vi "PWA_Setup_Panel.vi"(0 "Show Panel?":bool, 1 "Check Calib file?":bool, 2 "OK":T1, 3 "Incoming Setup String":string) -> (7 "Outgoing Setup String":string)   [LabVIEW 2017]
uses:
  Controls/ok_button.ctl
  File/Setup_Filetype.ctl
  Controls/Post_Process.ctl
  Controls/App_Global.ctl
  Controls/Inst_type.ctl
  Globals/Meas_global.vi
  PWAtasksGLOBAL.vi
panel:
  in  "Probe Rotated Thro' 180":bool
  in  "Software + buffering delay per pulse (s)":dbl=9.7e-06
  in  "Symbol":string
  in  "Pulse length \nx2 micro sec":i16=1 min=1 max=12
  in  "Clock Rate":bool
  in  "Gain":i16=1 min=1 max=12
  in  "Wire Current mA":i16(knob)=1 min=1 max=3 step=1 scale=1.0..3.0
  in  "Trigger -ve":dbl(knob)=1.0 min=0.0 max=5.0 scale=0.0..5.0 scale format="%#.2f"
  in  "Trigger +ve":dbl(knob)=1.0 min=0.0 max=5.0 scale=0.0..5.0 scale format="%#.2f"
  out "Calib Path from file":path
  in  "Use Latest":bool=TRUE
  in  "PWA Calib. File Path":path=path "/G5_1_HD/Users/paulhayden/Desktop/Labview test/PWA_Calib.xls"
  in  "Minimum TOF (mu.s)":i16=225
  in  "PWA Freq. (Hz)":dbl=30.0 min=0.0 max=50.0
  # "PELA Flow Instruments Ltd."
  # "TRIGGER LEVELS\n(volts)"
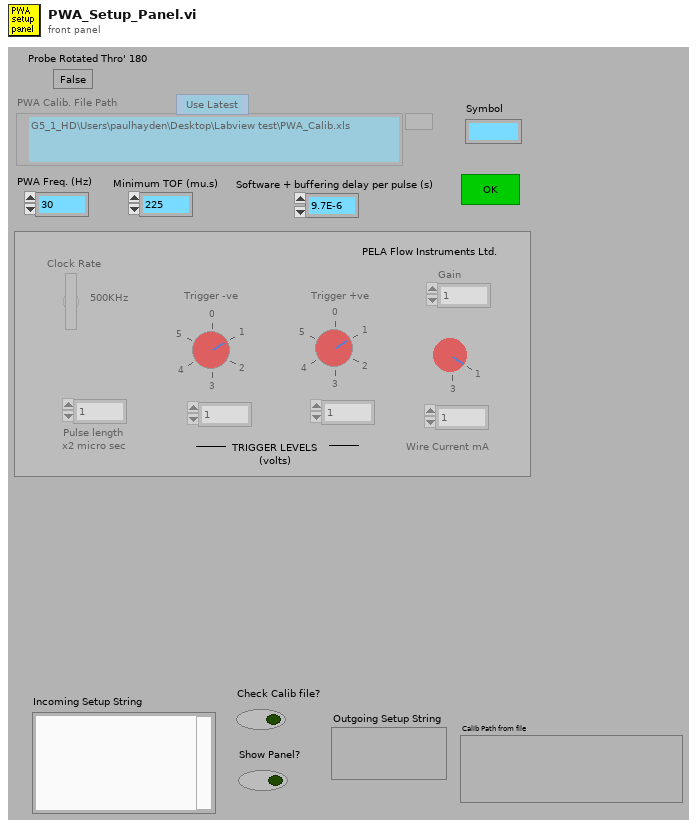
[diagram p1: front panel]
types:
  T1 = typedef "ok_button.ctl" = bool
  T2 = typedef "Setup_Filetype.ctl" = enum16{"Measurement Setups", "Calibration Setups", "General", "Results File Plotter Setups", "Speed Calib Tweaks"}
  T3 = typedef "Post_Process.ctl" = enum16{"Take New Data", "Post Process Raw Data File"}
  T4 = typedef "App_Global.ctl" = enum16{"Read Global", "Write to Global", "Initialise Array"}
  T5 = typedef "Inst_type.ctl" = enum16{"Propeller anemometer", "Raw voltage", "Pressure Transducer", "Pitot-static tube", "Preston tube", "Hot wire", "Cross wire 1", "Cross wire 2", "Generic Linear", "Generic Polynomial", "Generic BackPoly", "Fast FID", "Thermocouple", "Cold wire", "Pulsed Wire", "LDA Vel", "LDA Tran time", "LDA Arr time", "Microphone"}
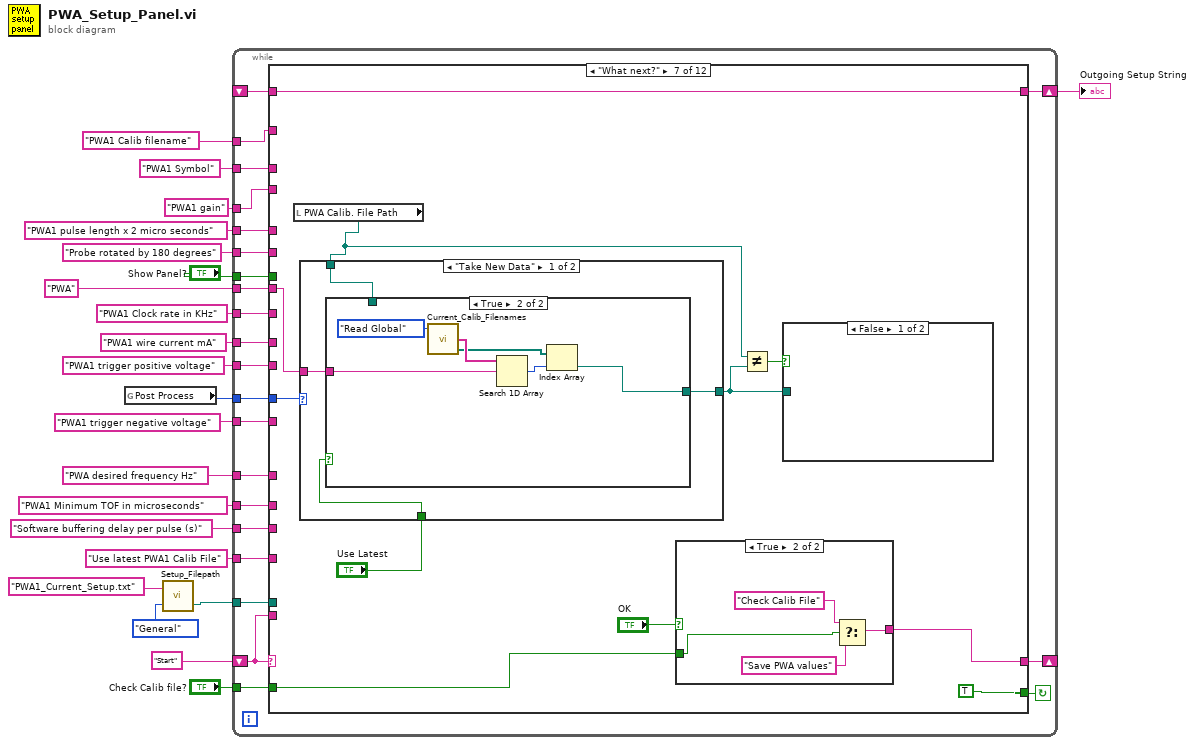
[diagram p0: block diagram]
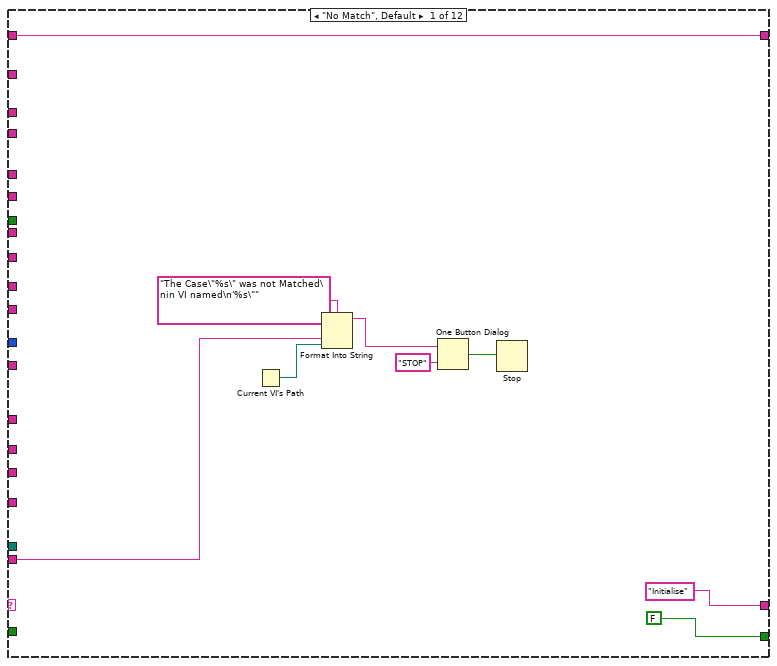
[diagram p2: hidden frame]
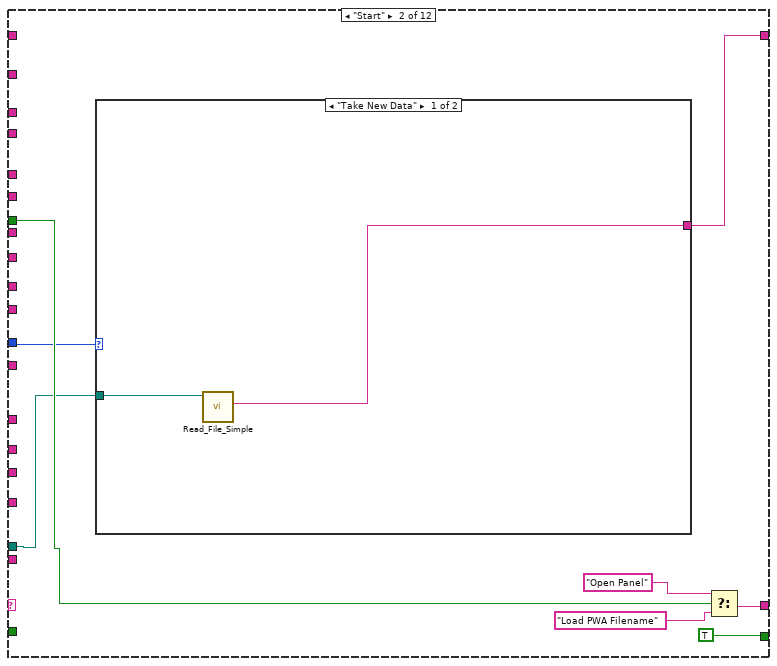
[diagram p3: hidden frame]
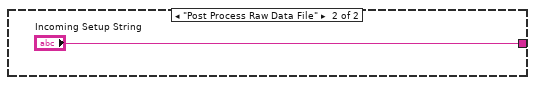
[diagram p4: hidden frame]
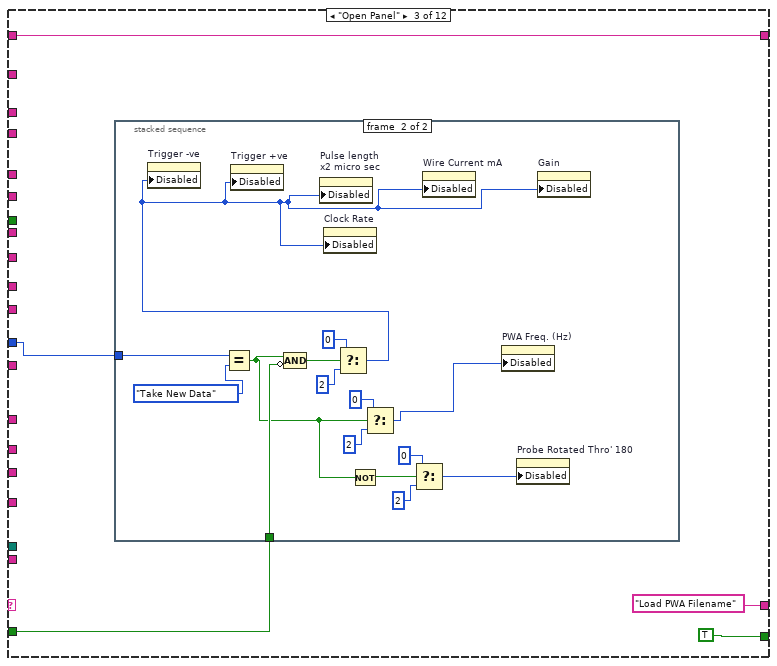
[diagram p5: hidden frame]
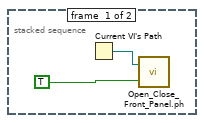
[diagram p6: hidden frame]
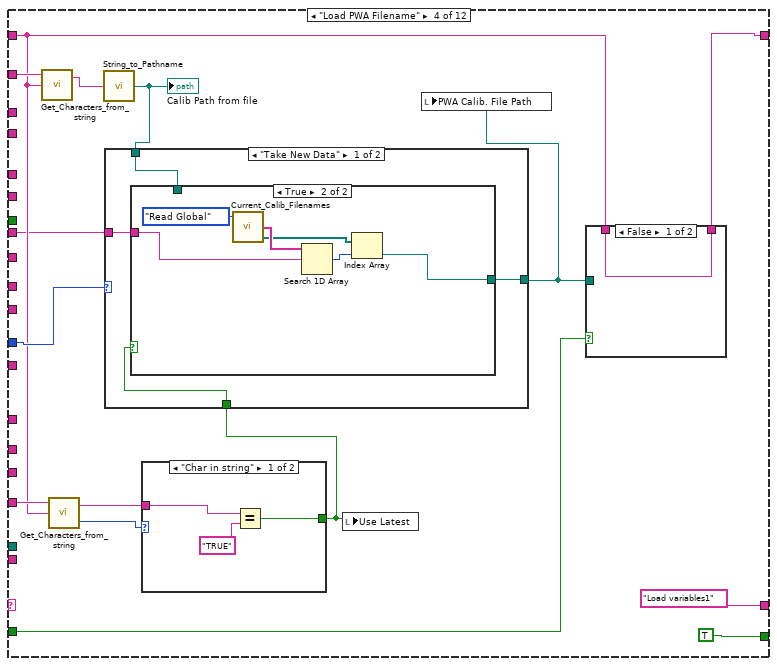
[diagram p7: hidden frame]
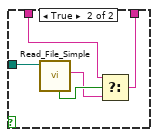
[diagram p8: hidden frame]
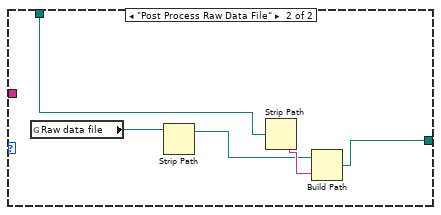
[diagram p10: hidden frame]
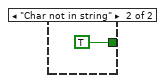
[diagram p11: hidden frame]
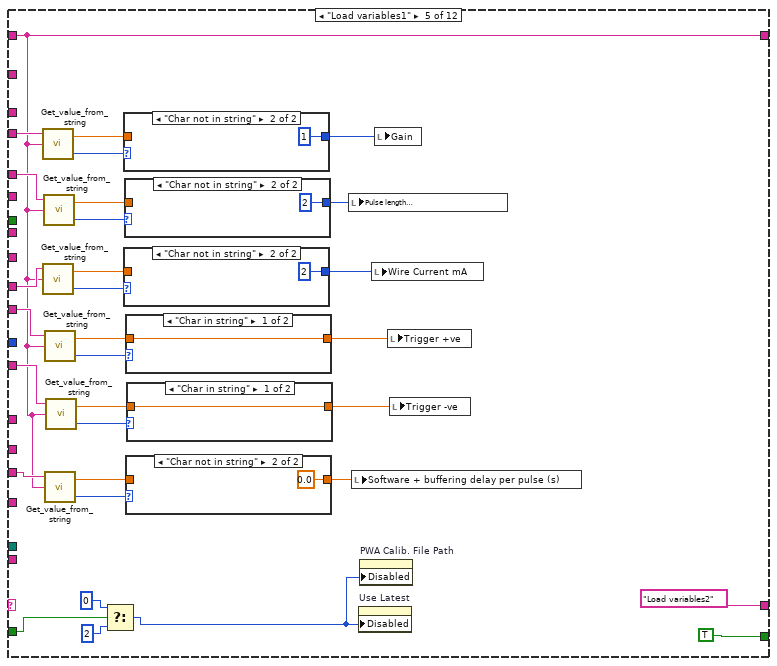
[diagram p12: hidden frame]
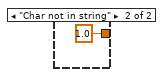
[diagram p14: hidden frame]
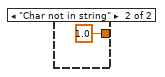
[diagram p15: hidden frame]
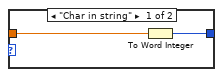
[diagram p16: hidden frame]
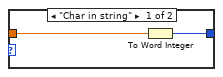
[diagram p17: hidden frame]
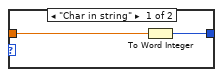
[diagram p18: hidden frame]
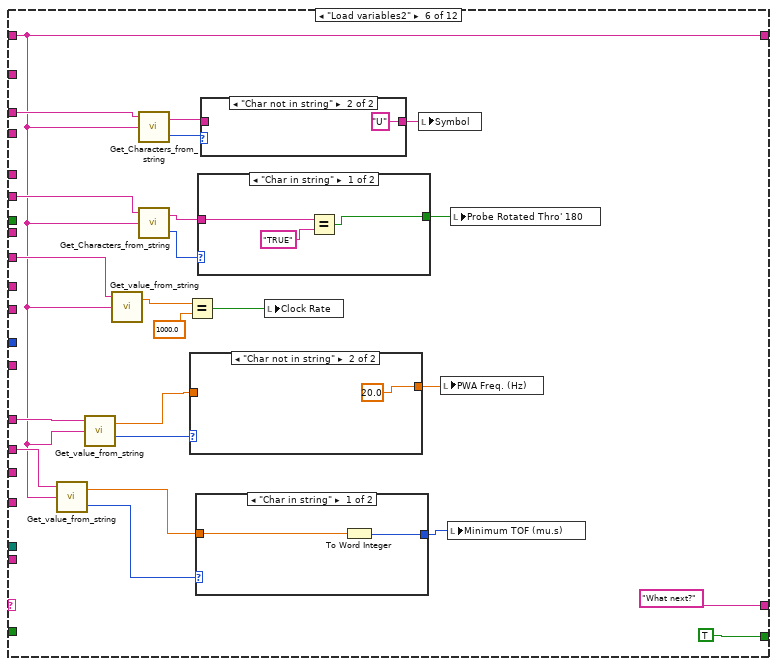
[diagram p19: hidden frame]
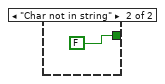
[diagram p20: hidden frame]
diagram:
  n1 = global read "Meas_global.vi" "Post Process"() -> (w20:T3)
  n2 = call "Setup_Filepath.vi"("Setup File Type"=Setup_Filetype."General", "Filename in"="PWA1_Current_Setup.txt" ("name or relative path")) -> ("Filename Out"=w2:path)  [unwired: 1 out]
  n3 = while {
    shift-left: "Start" -> [w43]
    shift-right: [w44] -> _
    tunnel: "Show Panel?" -> [w42]
    tunnel: w20 -> [w41]
    tunnel: "PWA1 Calib filename" -> [w39]
    tunnel: "Use latest PWA1 Calib File" -> [w40]
    tunnel: "PWA1 Minimum TOF in microseconds" -> [w38]
    tunnel: "PWA desired frequency Hz" -> [w37]
    tunnel: "Check Calib file?" -> [w36]
    tunnel: "PWA1 gain" -> [w35]
    tunnel: "PWA1 pulse length x 2 micro seconds" -> [w34]
    tunnel: "PWA1 wire current mA" -> [w33]
    tunnel: "PWA1 trigger positive voltage" -> [w32]
    tunnel: "PWA1 trigger negative voltage" -> [w31]
    tunnel: "PWA1 Clock rate in KHz" -> [w30]
    shift-right: [w29] -> w7
    shift-left: _ -> [w28]
    tunnel: "PWA1 Symbol" -> [w27]
    tunnel: w2 -> [w26]
    tunnel: "Software buffering delay per pulse (s)" -> [w25]
    tunnel: "Probe rotated by 180 degrees" -> [w24]
    tunnel: "PWA" ("element") -> [w23]
    stop <- w45 continue-if-true
    n4 = case shown="\"What next?\"" w43 {
      tunnel: [FALSE TRUE TRUE TRUE TRUE TRUE TRUE TRUE ("Show Panel?") TRUE ("Show Panel?") TRUE ("Show Panel?") w338 FALSE ("Show Panel?")] -> w45
      tunnel: ["Initialise" w55 "Load PWA Filename" "Load variables1" "Load variables2" "What next?" w216 "Save PWA values" "2nd Save PWA values" "PWA Setup Summary" "Close Panel" "End"] -> w44
      tunnel: w43 -> [w49 _ _ _ _ _ _ _ _ _ _ _]
      tunnel: w42 -> [_ w61 _ _ _ _ _ _ _ _ w338 _]
      tunnel: w41 -> [_ w58 w68 w94 _ _ w218 _ _ _ _ w340]
      tunnel: w40 -> [_ _ _ w96 _ _ _ _ w276 _ _ _]
      tunnel: w39 -> [_ _ _ w99 _ _ _ _ w286 _ _ _]
      tunnel: w38 -> [_ _ _ _ _ w195 _ _ w284 _ _ _]
      tunnel: w37 -> [_ _ _ _ _ w194 _ _ w285 _ _ _]
      tunnel: w36 -> [_ _ w66 w91 w157 _ w214 _ _ _ _ _]
      tunnel: w35 -> [_ _ _ _ w150 _ _ _ _ w323 _ _]
      tunnel: w34 -> [_ _ _ _ w146 _ _ _ _ w307 _ _]
      tunnel: w33 -> [_ _ _ _ w134 _ _ _ _ w312 _ _]
      tunnel: w32 -> [_ _ _ _ w139 _ _ _ _ w309 _ _]
      tunnel: w31 -> [_ _ _ _ w135 _ _ _ _ w308 _ _]
      tunnel: w30 -> [_ _ _ _ _ w187 _ _ _ w318 _ _]
      tunnel: [w46 w57 w67 w89 w130 w178 w213 w248 w272 w298 w328 w344] -> w29
      tunnel: w28 -> [w46 _ w67 w90 w130 w178 w213 w248 _ w299 w328 w344]
      tunnel: w27 -> [_ _ _ _ _ w183 _ _ w270 _ _ _]
      tunnel: w26 -> [_ w56 _ _ _ _ _ _ _ _ _ w343]
      tunnel: w25 -> [_ _ _ _ w131 _ _ _ _ w296 _ _]
      tunnel: w24 -> [_ _ _ _ _ w179 _ _ w263 _ _ _]
      tunnel: w23 -> [_ _ _ w88 _ _ w209 w243 _ _ _ _]
      frame "No Match", Default {
        n5 = Current VI's Path() -> (path=w48:path)
        n6 = Format Into String(format string="The Case\"%s\" was not Matched\nin VI named\n'%s\"" ("Format String"), w49, w48) -> (resulting string=w52:string)  [unwired: 2 in, 1 out]
        n7 = One Button Dialog(message=w52, button name ("OK")="STOP") -> (true=w50:bool)
        n8 = Stop(stop? (T)=w50) -> ()
      }
      frame "Start" {
        n9 = case shown="\"Take New Data\"" w58 {
          tunnel: [w63 "Incoming Setup String"] -> w57
          tunnel: w56 -> [w64 _]
          frame "Take New Data" {
            n10 = call "Read_File_Simple.vi"("Filename"=w64) -> ("string"=w63:string)  [unwired: 2 in, 7 out]
          }
          frame "Post Process Raw Data File" {
          }
        }
        n11 = Select(t="Open Panel", s=w61, f="Load PWA Filename") -> (s? t:f=w55:string)
      }
      frame "Open Panel" {
        n12 = stacked-sequence {
          tunnel: w68 -> [_ w87]
          tunnel: w66 -> [_ w82]
          frame #0 {
            n13 = Current VI's Path() -> (path=w72:path)
            n14 = call "Open_Close_Front_Panel.ph.vi"("Front Panel Window:Open"=TRUE, "VI path"=w72) -> ()  [unwired: 2 out]
          }
          frame #1 {
            n15 = Equal?(x=w87, y=Post_Process."Take New Data" ("Post Process")) -> (x = y?=w75:bool)
            n16 = Compound Arithmetic op=AND(w75, invert w82) -> (w81:bool)
            n17 = Select(t=u8 0 ("Disabled"), s=w81, f=u8 2) -> (s? t:f=w83:u8)
            n18 = property on="Trigger -ve" class="Knob (strict)"("Disabled"=w83) -> ()  [unwired: 2 in, 2 out]
            n19 = property on="Trigger +ve" class="Knob (strict)"("Disabled"=w83) -> ()  [unwired: 2 in, 2 out]
            n20 = property on="Pulse length \nx2 micro sec" class="DigNum (strict)"("Disabled"=w83) -> ()  [unwired: 2 in, 2 out]
            n21 = property on="Clock Rate" class="Bool (strict)"("Disabled"=w83) -> ()  [unwired: 2 in, 2 out]
            n22 = Not(x=w75) -> (.not. x?=w74:bool)
            n23 = Select(t=u8 0 ("Disabled"), s=w75, f=u8 2) -> (s? t:f=w78:u8)
            n24 = Select(t=u8 0 ("Disabled"), s=w74, f=u8 2) -> (s? t:f=w73:u8)
            n25 = property on="Wire Current mA" class="Knob (strict)"("Disabled"=w83) -> ()  [unwired: 2 in, 2 out]
            n26 = property on="PWA Freq. (Hz)" class="DigNum (strict)"("Disabled"=w78) -> ()  [unwired: 2 in, 2 out]
            n27 = property on="Probe Rotated Thro' 180" class="Bool (strict)"("Disabled"=w73) -> ()  [unwired: 2 in, 2 out]
            n28 = property on="Gain" class="DigNum (strict)"("Disabled"=w83) -> ()  [unwired: 2 in, 2 out]
          }
        }
      }
      frame "Load PWA Filename" {
        n29 = call "Get_Characters_from_string.vi"("Input string"=w90, "Variable name"=w99) -> ("Value"=w100:string)  [unwired: 1 in, 1 out]
        n30 = call "Get_Characters_from_string.vi"("Input string"=w90, "Variable name"=w96) -> ("Status"=w97:enum16{"Char in string", "Char not in string"}, "Value"=w98:string)  [unwired: 1 in]
        n31 = call "String_to_Pathname.vi"("Input String"=w100) -> ("path"=w95:path)
        "Calib Path from file" <- w95
        n32 = case shown="\"Char in string\"" w97 {
          tunnel: w98 -> [w127 _]
          tunnel: [w125 TRUE] -> w93
          frame "Char in string" {
            n33 = Equal?(x=w127, y="TRUE") -> (x = y?=w125:bool)
          }
          frame "Char not in string" {
          }
        }
        n34 = case shown="\"Take New Data\"" w94 {
          tunnel: [w111 w120] -> w92
          tunnel: w95 -> [w110 w123]
          tunnel: w93 -> [w112 _]
          tunnel: w88 -> [w109 _]
          frame "Take New Data" {
            n35 = case shown="True" w112 {
              tunnel: [w113 w115] -> w111
              tunnel: w110 -> [w113 _]
              tunnel: w109 -> [_ w114]
              frame False {
              }
              frame True {
                n36 = call "Current_Calib_Filenames.vi"("Mode"=App_Global."Read Global") -> ("Calib Filename Out"=w117:path[], "Channel ID Output"=w118:string[])  [unwired: 2 in, 1 out]
                n37 = Search 1D Array(1D array=w118, element=w114) -> (index of element=w116:i32)  [unwired: 1 out]
                n38 = Index Array(array=w117, index=w116) -> (element=w115:path)
              }
            }
          }
          frame "Post Process Raw Data File" {
            n39 = global read "Meas_global.vi" "Raw data file"() -> (w124:path)
            n40 = Strip Path(path=w124) -> (stripped path=w121:path)  [unwired: 1 out]
            n41 = Strip Path(path=w123) -> (name=w122:string)  [unwired: 1 out]
            n42 = Build Path(base path=w121, name or relative path=w122) -> (appended path=w120:path)
          }
        }
        n43 = local write "Use Latest"(w93) -> ()
        n44 = local write "PWA Calib. File Path"(w92) -> ()
        n45 = case shown="False" w91 {
          tunnel: w92 -> [_ w108]
          tunnel: w90 -> [w103 w105]
          tunnel: [w103 w104] -> w89
          frame False {
          }
          frame True {
            n46 = call "Read_File_Simple.vi"("Filename"=w108) -> ("Error?"=w107:bool, "string"=w106:string)  [unwired: 2 in, 6 out]
            n47 = Select(t=w105, s=w107, f=w106) -> (s? t:f=w104:string)
          }
        }
      }
      frame "Load variables1" {
        n48 = call "Get_value_from_string.vi"("Input string"=w130, "Variable name"=w150) -> ("Status"=w152:enum16{"Char in string", "Char not in string"}, "Value"=w153:dbl)  [unwired: 1 in]
        n49 = call "Get_value_from_string.vi"("Input string"=w130, "Variable name"=w134) -> ("Status"=w144:enum16{"Char in string", "Char not in string"}, "Value"=w145:dbl)  [unwired: 1 in]
        n50 = call "Get_value_from_string.vi"("Input string"=w130, "Variable name"=w146) -> ("Status"=w148:enum16{"Char in string", "Char not in string"}, "Value"=w147:dbl)  [unwired: 1 in]
        n51 = call "Get_value_from_string.vi"("Input string"=w130, "Variable name"=w139) -> ("Status"=w141:enum16{"Char in string", "Char not in string"}, "Value"=w140:dbl)  [unwired: 1 in]
        n52 = call "Get_value_from_string.vi"("Input string"=w130, "Variable name"=w131) -> ("Status"=w132:enum16{"Char in string", "Char not in string"}, "Value"=w129:dbl)  [unwired: 1 in]
        n53 = call "Get_value_from_string.vi"("Input string"=w130, "Variable name"=w135) -> ("Status"=w137:enum16{"Char in string", "Char not in string"}, "Value"=w138:dbl)  [unwired: 1 in]
        n54 = Select(t=u8 0 ("Disabled"), s=w157, f=u8 2 ("Disabled")) -> (s? t:f=w154:u8)
        n55 = case shown="\"Char not in string\"" w152 {
          tunnel: w153 -> [w173 _]
          tunnel: [w172 i16 1 ("PWA No. of Samples")] -> w151
          frame "Char in string" {
            n56 = To Word Integer(number=w173) -> (16bit integer=w172:i16)
          }
          frame "Char not in string" {
          }
        }
        n57 = case shown="\"Char not in string\"" w144 {
          tunnel: w145 -> [w167 _]
          tunnel: [w166 i16 2 ("PWA No. of Samples")] -> w143
          frame "Char in string" {
            n58 = To Word Integer(number=w167) -> (16bit integer=w166:i16)
          }
          frame "Char not in string" {
          }
        }
        n59 = case shown="\"Char not in string\"" w148 {
          tunnel: w147 -> [w170 _]
          tunnel: [w169 i16 2 ("PWA No. of Samples")] -> w149
          frame "Char in string" {
            n60 = To Word Integer(number=w170) -> (16bit integer=w169:i16)
          }
          frame "Char not in string" {
          }
        }
        n61 = case shown="\"Char in string\"" w141 {
          tunnel: w140 -> [w164 _]
          tunnel: [w164 1.0 ("Value")] -> w142
          frame "Char in string" {
          }
          frame "Char not in string" {
          }
        }
        n62 = case shown="\"Char not in string\"" w132 {
          tunnel: w129 -> [w160 _]
          tunnel: [w160 0.0 ("Value")] -> w133
          frame "Char in string" {
          }
          frame "Char not in string" {
          }
        }
        n63 = case shown="\"Char in string\"" w137 {
          tunnel: w138 -> [w162 _]
          tunnel: [w162 1.0 ("Value")] -> w136
          frame "Char in string" {
          }
          frame "Char not in string" {
          }
        }
        n64 = local write "Pulse length \nx2 micro sec"(w149) -> ()
        n65 = local write "Software + buffering delay per pulse (s)"(w133) -> ()
        n66 = property on="Use Latest" class="Bool (strict)"("Disabled"=w154) -> ()  [unwired: 2 in, 2 out]
        n67 = property on="PWA Calib. File Path" class="Path"("Disabled"=w154) -> ()  [unwired: 2 in, 2 out]
        n68 = local write "Wire Current mA"(w143) -> ()
        n69 = local write "Gain"(w151) -> ()
        n70 = local write "Trigger +ve"(w142) -> ()
        n71 = local write "Trigger -ve"(w136) -> ()
      }
      frame "Load variables2" {
        n72 = call "Get_value_from_string.vi"("Input string"=w178, "Variable name"=w195) -> ("Status"=w190:enum16{"Char in string", "Char not in string"}, "Value"=w189:dbl)  [unwired: 1 in]
        n73 = call "Get_value_from_string.vi"("Input string"=w178, "Variable name"=w194) -> ("Status"=w193:enum16{"Char in string", "Char not in string"}, "Value"=w192:dbl)  [unwired: 1 in]
        n74 = call "Get_value_from_string.vi"("Input string"=w178, "Variable name"=w187) -> ("Value"=w186:dbl)  [unwired: 1 in, 1 out]
        n75 = call "Get_Characters_from_string.vi"("Input string"=w178, "Variable name"=w183) -> ("Status"=w182:enum16{"Char in string", "Char not in string"}, "Value"=w181:string)  [unwired: 1 in]
        n76 = call "Get_Characters_from_string.vi"("Input string"=w178, "Variable name"=w179) -> ("Status"=w177:enum16{"Char in string", "Char not in string"}, "Value"=w175:string)  [unwired: 1 in]
        n77 = Equal?(x=w186, y=1000.0) -> (x = y?=w184:bool)
        n78 = case shown="\"Char not in string\"" w193 {
          tunnel: w192 -> [w207 _]
          tunnel: [w207 20.0 ("PWA No. of Samples")] -> w191
          frame "Char in string" {
          }
          frame "Char not in string" {
          }
        }
        n79 = case shown="\"Char in string\"" w190 {
          tunnel: w189 -> [w205 _]
          tunnel: [w204 i16 225 ("Minimum TOF (mu.s)")] -> w188
          frame "Char in string" {
            n80 = To Word Integer(number=w205) -> (16bit integer=w204:i16)
          }
          frame "Char not in string" {
          }
        }
        n81 = case shown="\"Char in string\"" w177 {
          tunnel: [w198 FALSE] -> w176
          tunnel: w175 -> [w200 _]
          frame "Char in string" {
            n82 = Equal?(x=w200, y="TRUE") -> (x = y?=w198:bool)
          }
          frame "Char not in string" {
          }
        }
        n83 = case shown="\"Char not in string\"" w182 {
          tunnel: w181 -> [w202 _]
          tunnel: [w202 "U" ("Value")] -> w180
          frame "Char in string" {
          }
          frame "Char not in string" {
          }
        }
        n84 = local write "Clock Rate"(w184) -> ()
        n85 = local write "Symbol"(w180) -> ()
        n86 = local write "PWA Freq. (Hz)"(w191) -> ()
        n87 = local write "Minimum TOF (mu.s)"(w188) -> ()
        n88 = local write "Probe Rotated Thro' 180"(w176) -> ()
      }
      frame "What next?" {
        n89 = local read "PWA Calib. File Path"() -> (w212:path)
        n90 = case shown="\"Take New Data\"" w218 {
          tunnel: [w229 w238] -> w210
          tunnel: w212 -> [w228 w241]
          tunnel: "Use Latest" -> [w230 _]
          tunnel: w209 -> [w227 _]
          frame "Take New Data" {
            n91 = case shown="True" w230 {
              tunnel: [w231 w233] -> w229
              tunnel: w228 -> [w231 _]
              tunnel: w227 -> [_ w232]
              frame False {
              }
              frame True {
                n92 = call "Current_Calib_Filenames.vi"("Mode"=App_Global."Read Global") -> ("Calib Filename Out"=w235:path[], "Channel ID Output"=w236:string[])  [unwired: 2 in, 1 out]
                n93 = Search 1D Array(1D array=w236, element=w232) -> (index of element=w234:i32)  [unwired: 1 out]
                n94 = Index Array(array=w235, index=w234) -> (element=w233:path)
              }
            }
          }
          frame "Post Process Raw Data File" {
            n95 = global read "Meas_global.vi" "Raw data file"() -> (w242:path)
            n96 = Strip Path(path=w242) -> (stripped path=w239:path)  [unwired: 1 out]
            n97 = Strip Path(path=w241) -> (name=w240:string)  [unwired: 1 out]
            n98 = Build Path(base path=w239, name or relative path=w240) -> (appended path=w238:path)
          }
        }
        n99 = case shown="True" "OK" {
          tunnel: ["What next?" ("f") w224] -> w216
          tunnel: w214 -> [_ w223]
          frame False {
            n100 = Wait (ms)(milliseconds to wait=u32 300) -> ()  [unwired: 1 out]
          }
          frame True {
            n101 = Select(t="Check Calib File", s=w223, f="Save PWA values") -> (s? t:f=w224:string)
          }
        }
        n102 = Not Equal?(x=w212, y=w210) -> (x != y?=w211:bool)
        n103 = case shown="False" w211 {
          tunnel: w210 -> [_ w220]
          frame False {
          }
          frame True {
            n104 = local write "PWA Calib. File Path"(w220) -> ()
          }
        }
      }
      frame "Check Calib File" {
        n105 = local read "Use Latest"() -> (w244:bool)
        n106 = local read "PWA Calib. File Path"() -> (w247:path)
        n107 = call "Find_calibration_file.vi"("Inst type"=Inst_type."Pulsed Wire", "Use Latest Calib"=w244, "filename"=w247) -> ("filename out"=w246:path)  [unwired: 1 in]
        n108 = Not Equal?(x=w246, y=w247) -> (x != y?=w250:bool)
        n109 = And(x=w250, y=w244) -> (x .and. y?=w249:bool)
        n110 = local write "PWA Calib. File Path"(w246) -> ()
        n111 = case shown="True" w249 {
          tunnel: w246 -> [_ w254]
          tunnel: w243 -> [_ w253]
          frame False {
          }
          frame True {
            n112 = Build Array(w254) -> (w257:path[])
            n113 = Build Array(w253) -> (w256:string[])
            n114 = call "Current_Calib_Filenames.vi"("Calib Filename"=w257, "Channel ID input"=w256, "Mode"=App_Global."Write to Global") -> ()  [unwired: 3 out]
          }
        }
      }
      frame "Save PWA values" {
        n115 = local read "Use Latest"() -> (w280:bool)
        n116 = global write "PWAtasksGLOBAL.vi" "PWA Freq. (Hz)"("PWA Freq. (Hz)") -> ()
        n117 = global write "PWAtasksGLOBAL.vi" "PWA Calib. File Path"("PWA Calib. File Path") -> ()
        n118 = Select(t="TRUE", s=w280, f="FALSE") -> (s? t:f=w277:string)
        n119 = global write "PWAtasksGLOBAL.vi" "PWA Symbol"("Symbol") -> ()
        n120 = call "Characters_to_string.vi"("Characters to write"="Symbol", "Label for characters"=w270) -> ("Output string"=w269:string)
        n121 = call "Characters_to_string.vi"("Characters to write"=w277, "Label for characters"=w276) -> ("Output string"=w275:string)
        n122 = call "Value_to_string.vi"("Value"="PWA Freq. (Hz)", "Label for value"=w285) -> ("Output string"=w282:string)  [unwired: 1 in]
        n123 = global write "PWAtasksGLOBAL.vi" "Probe Rotated Thro' 180"("Probe Rotated Thro' 180") -> ()
        n124 = call "Path_2_String.vi"("Real Path"="PWA Calib. File Path") -> ("Path String"=w287:string)
        n125 = Select(t="TRUE" ("y"), s="Probe Rotated Thro' 180", f="FALSE") -> (s? t:f=w259:string)
        n126 = call "Characters_to_string.vi"("Characters to write"=w259, "Label for characters"=w263) -> ("Output string"=w260:string)
        n127 = call "Characters_to_string.vi"("Characters to write"=w287, "Label for characters"=w286) -> ("Output string"=w283:string)
        n128 = local read "Clock Rate"() -> (w267:bool)
        n129 = case shown="True" w267 {
          tunnel: [w290 w294] -> w266
          tunnel: [w289 w294] -> w265
          tunnel: "Minimum TOF (mu.s)" -> [w292 w294]
          frame False {
            w291 = i16 2 ("y")
            n130 = Divide(x=w292, y=w291) -> (x/y=w293:dbl)
            n131 = To Word Integer(number=w293) -> (16bit integer=w290:i16)
            n132 = Multiply(x=w290, y=w291) -> (x*y=w289:i16)
          }
          frame True {
          }
        }
        n133 = call "Value_to_string.vi"("Value"=w265, "Label for value"=w284) -> ("Output string"=w281:string)  [unwired: 1 in]
        n134 = Concatenate Strings(w283, w269, w260, w282, w281, w275) -> (w272:string)
        n135 = global write "PWAtasksGLOBAL.vi" "Minimum TOF Index"(w266) -> ()
      }
      frame "2nd Save PWA values" {
        n136 = Select(t=1000.0, s="Clock Rate", f=500.0) -> (s? t:f=w317:dbl)
        n137 = call "Value_to_string.vi"("Value"="Gain", "Label for value"=w323) -> ("Output string"=w305:string)  [unwired: 1 in]
        n138 = call "Value_to_string.vi"("Value"="Trigger -ve", "Label for value"=w308) -> ("Output string"=w300:string)  [unwired: 1 in]
        n139 = call "Value_to_string.vi"("Value"="Wire Current mA", "Label for value"=w312) -> ("Output string"=w302:string)  [unwired: 1 in]
        n140 = call "Value_to_string.vi"("Value"="Trigger +ve", "Label for value"=w309) -> ("Output string"=w301:string)  [unwired: 1 in]
        n141 = call "Value_to_string.vi"("Value"="Pulse length \nx2 micro sec", "Label for value"=w307) -> ("Output string"=w304:string)  [unwired: 1 in]
        n142 = call "Value_to_string.vi"("Value"=w317, "Label for value"=w318) -> ("Output string"=w303:string)  [unwired: 1 in]
        n143 = Multiply(x=w317, y=1000.0) -> (x*y=w315:dbl)
        n144 = Reciprocal(x=w315) -> (1/x=w314:dbl)
        n145 = call "Value_to_string.vi"("Value"="Software + buffering delay per pulse (s)", "Label for value"=w296) -> ("Output string"=w295:string)  [unwired: 1 in]
        n146 = global write "PWAtasksGLOBAL.vi" "PWA Seconds per clock pulse"(w314) -> ()
        n147 = Concatenate Strings(w299, w305, w304, w303, w302, w301, w300, w295) -> (w298:string)
      }
      frame "PWA Setup Summary" {
        n148 = local read "Pulse length \nx2 micro sec"() -> (w333:i16)
        n149 = local read "Wire Current mA"() -> (w332:i16)
        n150 = local read "Clock Rate"() -> (w337:bool)
        n151 = local read "Trigger -ve"() -> (w335:dbl)
        n152 = local read "Trigger +ve"() -> (w334:dbl)
        n153 = local read "Gain"() -> (w331:i16)
        n154 = Select(t="1MHz", s=w337, f="500KHz") -> (s? t:f=w336:string)
        n155 = Format Into String(format string="Clock=%s; Trig -ve=%.2f; Trig +ve=%.2f; Pulse length=%dx2micro sec; wire current=%dmA; Gain=%d", w336, w335, w334, w333, w332, w331) -> (resulting string=w329:string)  [unwired: 2 in, 1 out]
        n156 = global write "PWAtasksGLOBAL.vi" "PWA Setup summary"(w329) -> ()
      }
      frame "Close Panel" {
        n157 = case shown="\"Take New Data\"" w340 {
          tunnel: w344 -> [w349 _]
          tunnel: w343 -> [w348 _]
          frame "Take New Data" {
            w347 = FALSE  # append to file? (new file:F)
            n158 = call "Write_File_Simple.vi"("append to file? (new file:F)"=w347, "character string"=w349, "file path"=w348) -> ()  [unwired: 2 out]
          }
          frame "Post Process Raw Data File" {
          }
        }
        n159 = Current VI's Path() -> (path=w342:path)
        n160 = call "Open_Close_Front_Panel.ph.vi"("Front Panel Window:Open"=FALSE, "VI path"=w342) -> ()  [unwired: 2 out]
      }
    }
  }
  "Outgoing Setup String" <- w7
